vi "Tree Strings.vi"(8 "error in (no error)":errorcluster, 11 "BetterItem in":refnum<class "BetterItem.lvclass">) -> (0 "error out":errorcluster, 1 "Child Text":string[](array[string]), 2 "Left Cell String":string, 3 "BetterItem out":refnum<class "BetterItem.lvclass">, 5 "Child Tag":string)   [LabVIEW 2020, in "BetterDragAndDrop.lvlib" / "BetterItem.lvclass"]
uses:
  BetterItem.lvclass
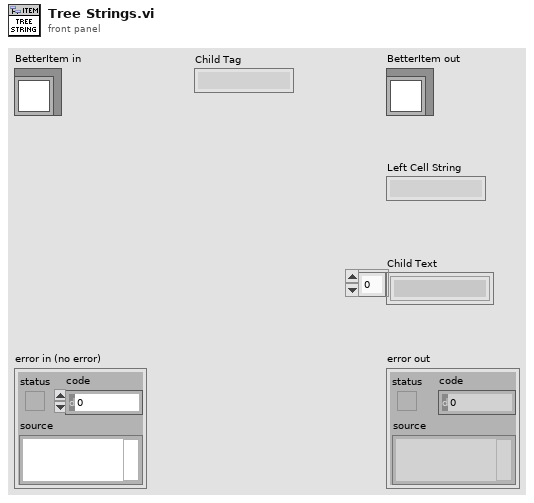
[diagram p1: front panel]
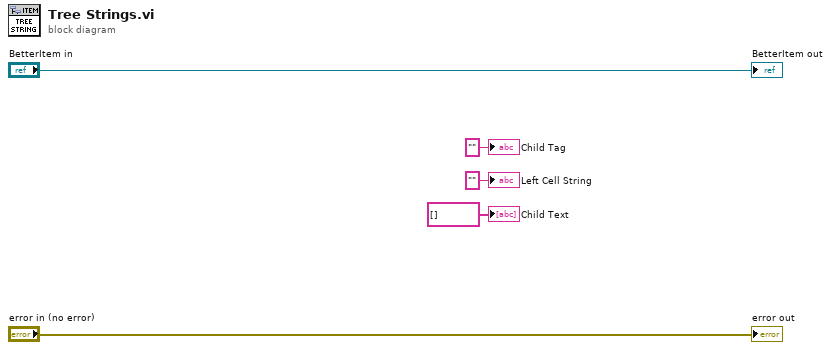
[diagram p0: block diagram]
diagram:
  "error out" <- "error in (no error)"
  "BetterItem out" <- "BetterItem in"
  "Left Cell String" <- "" ("Left Cell String")
  "Child Text" <- string[] [] ("Child Text")
  "Child Tag" <- "" ("Child Tag")
